vi "tst.vi"() -> ()   [LabVIEW 2021]
uses:
  C:/Localdata/Projects/TriekselSoft/TriekselsoftApplicationFramework/Source/.Externals/Library_EmguCV/Emgu.CV.Platform.NetStandard.dll
  Emgu.CV.Platform.NetStandard.dll
  <vilib>/picture/picture.llb/Draw True-Color Pixmap.vi
panel:
  in  "Numeric":dbl
  in  "stop":bool
  out "new picture":picture
  out "variant":variant
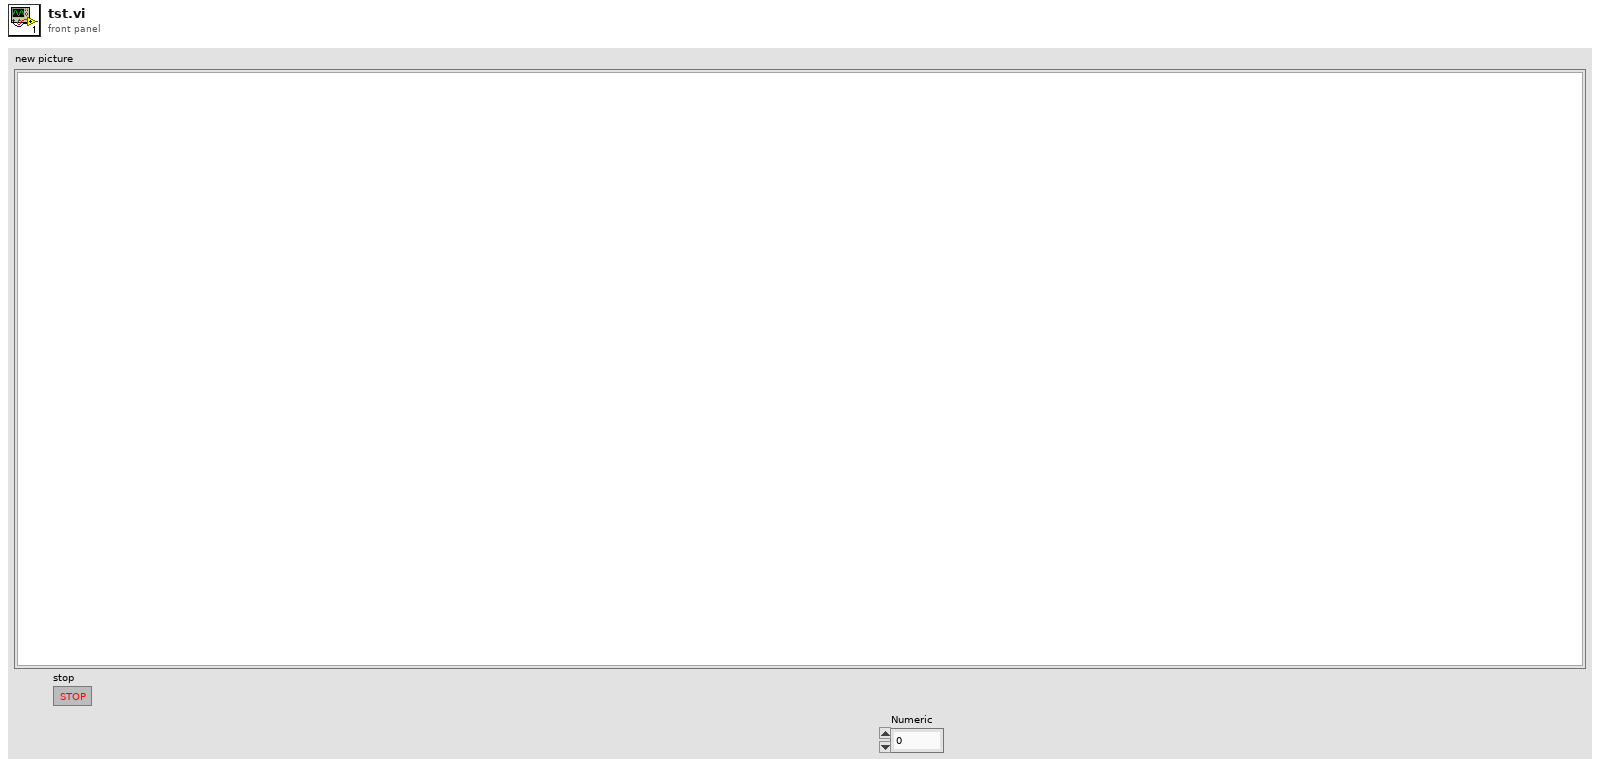
[diagram p1: front panel]
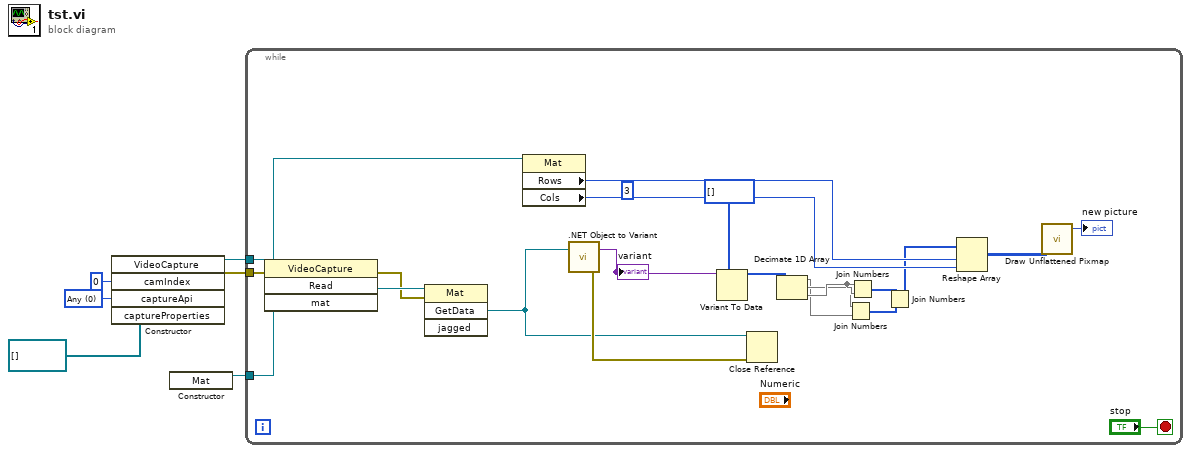
[diagram p0: block diagram]
diagram:
  w6 = 0 items=["Any"=0, "Vfw, V4L, V4L2"=200, "Firewire, IEEE1394, DC1394, CMU1394"=300, "QT"=500, "Unicap"=600, "DShow"=700, "Pvapi"=800, "OpenNI"=900, "OpenNIAsus"=910, "Android"=1000, "XiApi"=1100, "AVFoundation"=1200, "Giganetix"=1300, "Msmf"=1400, "Winrt"=1410, "IntelPerc"=1500, "Openni2"=1600, "Openni2Asus"=1610, "Gphoto2"=1700, "Gstreamer"=1800, "Ffmpeg"=1900, "Images"=2000, "Aravis"=2100, "OpencvMjpeg"=2200, "IntelMfx"=2300, "Xine"=2400] ("captureApi")
  n1 = constructor class="VideoCapture"("camIndex"=0, "captureApi"=w6, "captureProperties"=refnum<k24>[] []) -> (reference out=w3:refnum<k24>, error out=w2:errorcluster)  [unwired: 3 in, 4 out]
  n2 = constructor class="Mat"() -> (reference out=w1:refnum<k24>)  [unwired: 3 in, 2 out]
  n3 = while {
    tunnel: w3 -> [w26]
    tunnel: w2 -> [w25]
    tunnel: w1 -> [w8]
    stop <- "stop" stop-if-true
    (unwired) 3 ("y")
    n4 = invoke class="VideoCapture" method="Read"(reference=w26, error in=w25, "mat"=w8) -> (error out=w7:errorcluster)  [unwired: 1 in, 3 out]
    n5 = invoke class="Mat" method="GetData"(reference=w8, error in=w7) -> ("GetData"=w17:refnum<k24>)  [unwired: 2 in, 3 out]
    n6 = property class="Mat"(reference=w8) -> ("Rows"=w21:i32, "Cols"=w20:i32)  [unwired: 1 in, 2 out]
    n7 = call <vilib>:".NET Object to Variant.vi"(".NET object"=w17) -> ("error out"=w18:errorcluster, "variant"=w24:variant)  [unwired: 1 in]
    "variant" <- w24
    n8 = Variant To Data(type=u8[] [], Variant=w24) -> (data=w19:u8[])  [unwired: 1 in, 1 out]
    n9 = Close Reference(reference=w17, error in (no error)=w18) -> ()  [unwired: 1 out]
    n10 = Decimate 1D Array(w19) -> (w9:u8[], w10:u8[], w11:u8[])
    n11 = Join Numbers(hi=w10, lo=w9) -> ((hi.lo)=w14:u16[])
    n12 = Join Numbers(hi=w11, lo=w11) -> ((hi.lo)=w15:u16[])
    n13 = Join Numbers(hi=w15, lo=w14) -> ((hi.lo)=w13:u32[])
    n14 = Reshape Array(w13, w21, w20) -> (w12:u32[][])
    n15 = call-poly <vilib>:"Draw Unflattened Pixmap.vi"("data (RGB format)"=w12) -> ("new picture"=→"new picture":picture)  [unwired: 8 in]
  }
